vi "Write Event to File.vi"(8 "error in (no error)":errorcluster, 10 "Event":T1={"Time Stamp"=timestamp(0 s since 1904-01-01), "Event Level"=enum."Info", "Context"="", "Message"="", "Error"={"status"=FALSE, "code"=0, "source"=""}, "Node"=""}, 11 "Event Reporter Module in":refnum<class "Event Reporter Module.lvclass">) -> (0 "error out":errorcluster, 3 "Event Reporter Module out":refnum<class "Event Reporter Module.lvclass">)   [LabVIEW 2020, in "Volatus.lvlib" / "Event Reporter Module.lvclass"]
uses:
  Event Reporter Module.lvclass
  Event.ctl
  Event Level.ctl
  lv-cdm/CDM-Config/ISO8601 Config.ctl
  lv-cdm/CDM-Config/Format.ctl
  lv-cdm/CDM-Config/Precision.ctl
  lv-cdm/CDM-Config/Timezone.ctl
  Event Reporter Module.lvclass/Event Reporter Module.ctl
  lv-cdm/CDM-Config/ISO-8601 Format Strings.vi
  lv-cdm/CDM-Config/CDM-Config.lvlib
  Volatus.lvlib
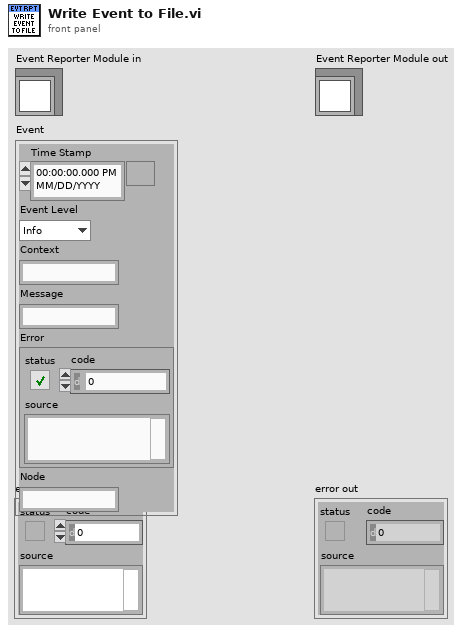
[diagram p1: front panel]
types:
  T1 = typedef "Volatus.lvlib/Event.ctl" = cluster{"Time Stamp":timestamp, "Event Level":T2, "Context":string, "Message":string, "Error":errorcluster, "Node":string}
  T2 = typedef "Volatus.lvlib/Event Level.ctl" = enum16{"Debug", "Info", "Warning", "Error"}
  T3 = typedef "CDM-Config.lvlib/ISO8601 Config.ctl" = cluster{"Format":T4, "Precision":T5, "Timezone":T6}
  T4 = typedef "CDM-Config.lvlib/Format.ctl" = enum16{"Extended", "Basic"}
  T5 = typedef "CDM-Config.lvlib/Precision.ctl" = enum16{"Millisecond", "Second", "Minute", "Hour", "Day"}
  T6 = typedef "CDM-Config.lvlib/Timezone.ctl" = enum16{"UTC", "Local"}
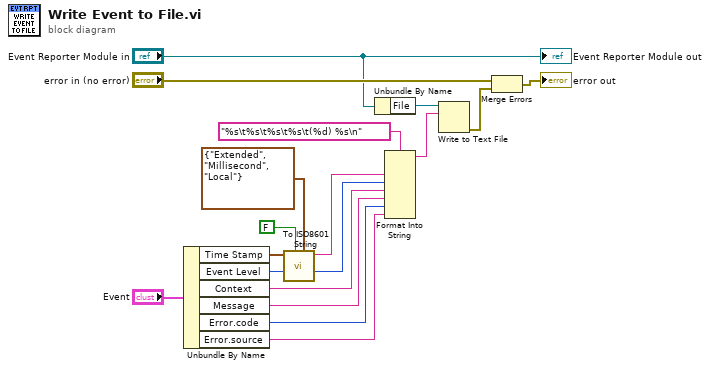
[diagram p0: block diagram]
diagram:
  n1 = Unbundle By Name("Event") -> ("Time Stamp"=w15:timestamp, "Event Level"=w11:T2, "Context"=w10:string, "Message"=w9:string, "Error.code"=w8:i32, "Error.source"=w7:string)
  n2 = call "To ISO8601 String.vi"("Format Config"=T3 {"Format"=enum."Extended", "Precision"=enum."Millisecond", "Timezone"=enum."Local"}, "Now for Unset? (T)"=FALSE, "Time Stamp"=w15) -> ("ISO 8601"=w12:string)  [unwired: 8 in]
  n3 = Unbundle By Name("Event Reporter Module in") -> ("File"=w4:refnum<file>)
  n4 = Format Into String(format string="%s\t%s\t%s\t%s\t(%d) %s\n", w12, w11, w10, w9, w8, w7) -> (resulting string=w3:string)  [unwired: 2 in, 1 out]
  n5 = Write to Text File(file (use dialog)=w4, text=w3) -> (error out=w1:errorcluster)  [unwired: 2 in, 2 out]
  n6 = Merge Errors("error in (no error)", w1) -> (→"error out":errorcluster)
  "Event Reporter Module out" <- "Event Reporter Module in"
